vi "Test JSON to Variant with JSON classes embedded.vi"() -> ()   [LabVIEW 2011]
uses:
  JSON Scalar/JSON Scalar.lvclass
  JSON Array/JSON Array.lvclass
  JSON Value/JSON Value.lvclass
  Variant JSON.lvlib
panel:
  out "String 2":string
  out "String":string
  out "x = y?":bool
  out "data":T1
  in  "Test Cluster":T1={"T2"="test2", "T1"=456.789, "Nest"={"Enum"=enum."AAA", "NestNest"={"A"="Hi", "B"=2.0, "C"=1.0+4.1i}}, "Test Array"=[456.789, 2.0, 3.0], "Boolean"=FALSE, "JSON Scalar"=refnum, "JSON Array"=refnum}
  out "JSON String":string
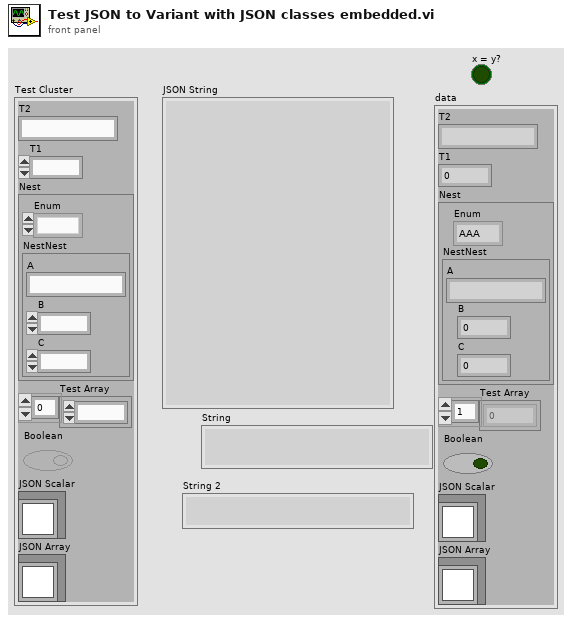
[diagram p1: front panel]
types:
  T1 = cluster{"T2":string, "T1":dbl, "Nest":cluster{"Enum":enum16{"AAA", "BBB", "CCC"}, "NestNest":cluster{"A":string, "B":dbl, "C":cdb}}, "Test Array":dbl[], "Boolean":bool, "JSON Scalar":refnum<class "JSON Scalar.lvclass">, "JSON Array":refnum<class "JSON Array.lvclass">}
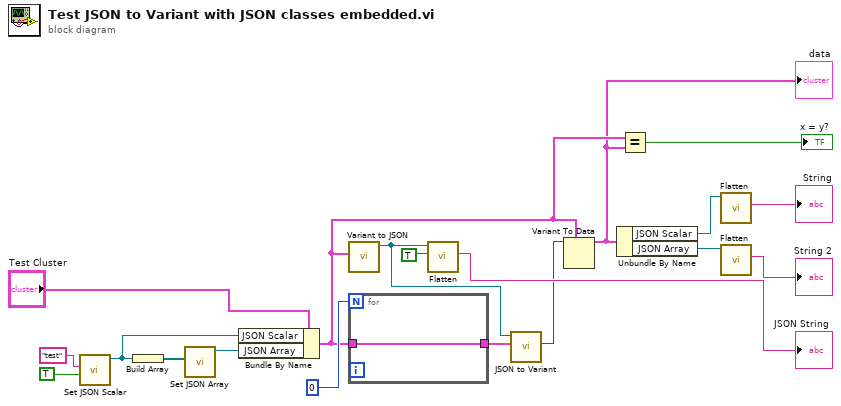
[diagram p0: block diagram]
diagram:
  n1 = call "Set JSON Scalar.vi"("Set as a JSON string (F)"=TRUE, "LabVIEW Text"="test") -> ("JSON Scalar out"=w5:refnum<class "JSON Scalar.lvclass">)  [unwired: 8 in, 1 out]
  n2 = Build Array(w5) -> (w4:refnum<class "JSON Scalar.lvclass">[])
  n3 = call "Set JSON Array.vi"("Array"=w4) -> ("JSON Array out"=w3:refnum<class "JSON Array.lvclass">)  [unwired: 9 in, 1 out]
  n4 = Bundle By Name(cluster="Test Cluster", "JSON Scalar"=w5, "JSON Array"=w3) -> (w9:T1)
  n5 = call "Variant to JSON.vi"("Variant"=w9) -> ("JSON Value out"=w17:refnum<class "JSON Value.lvclass">)  [unwired: 9 in, 1 out]
  n6 = for {
    N: 0 -> [_]
    tunnel: w9 -> [w20]
    tunnel: [w20] -> w13
  }
  n7 = call-dynamic "Flatten.vi"("Pretty Print?"=TRUE, "JSON Value in"=w17) -> ("String"=→"JSON String":string)  [unwired: 8 in, 1 out]
  n8 = call "JSON to Variant.vi"("Variant (Data Type)"=w13, "JSON Value"=w17) -> ("Variant out"=w16:variant)  [unwired: 8 in, 1 out]
  n9 = Variant To Data(type=w9, Variant=w16) -> (data=w8:T1)  [unwired: 1 in, 1 out]
  "data" <- w8
  n10 = Unbundle By Name(w8) -> ("JSON Scalar"=w7:refnum<class "JSON Scalar.lvclass">, "JSON Array"=w2:refnum<class "JSON Array.lvclass">)
  n11 = Equal?(x=w9, y=w8) -> (x = y?=→"x = y?":bool)
  n12 = call-dynamic "Flatten.vi"("JSON Scalar in"=w7) -> ("String"=→"String":string)  [unwired: 9 in, 1 out]
  n13 = call-dynamic "Flatten.vi"("JSON Array in"=w2) -> ("String"=→"String 2":string)  [unwired: 9 in, 1 out]
